vi "Sub VI TimeTest.vi"() -> ()   [LabVIEW 2021]
panel:
  out "ms / Cycle":dbl format="%.4f"
  in  "# Iterations":u32=10000
  in  "Device":T1(ring)
  in  "Instrument Address":refnum<visa-resource-name>
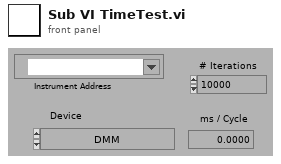
[diagram p1: front panel]
types:
  T1 = enum16{"DMM", "Keithley 2000", "HP 34401", "Memory Stats", "polynomial eval", "Null SubVI"}
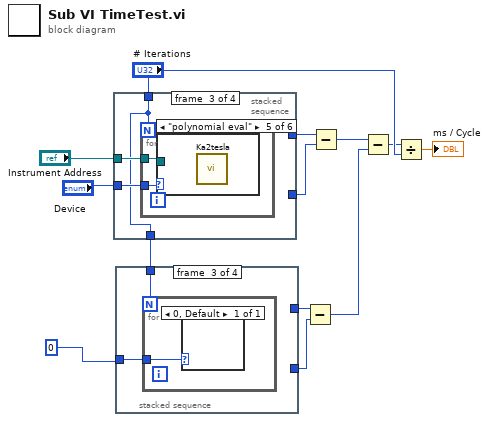
[diagram p0: block diagram]
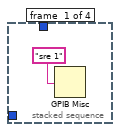
[diagram p2: hidden frame]
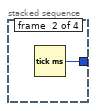
[diagram p3: hidden frame]
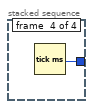
[diagram p4: hidden frame]
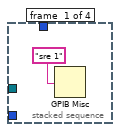
[diagram p5: hidden frame]
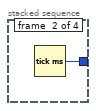
[diagram p6: hidden frame]
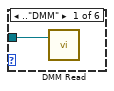
[diagram p7: hidden frame]
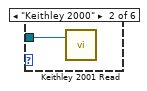
[diagram p8: hidden frame]
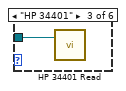
[diagram p9: hidden frame]
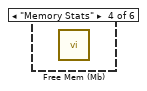
[diagram p10: hidden frame]
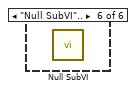
[diagram p11: hidden frame]
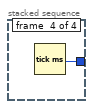
[diagram p12: hidden frame]
diagram:
  n1 = stacked-sequence {
    tunnel: "Instrument Address" -> [_ _ w18 _]
    tunnel: "Device" -> [_ _ w17 _]
    tunnel: "# Iterations" -> [_ _ w16 _]
    tunnel: [_ _ _ w24] -> w10
    tunnel: [_ w15 _ _] -> w9
    tunnel: [_ _ w16 _] -> w6
    frame #0 {
      n2 = GPIB Misc(0:"sre 1") -> ()  [unwired: 1 in, 3 out]
    }
    frame #1 {
      n3 = Tick Count (ms)() -> (millisecond timer value=w15:u32)
    }
    frame #2 {
      n4 = for {
        N: w16 -> [_]
        tunnel: w18 -> [w20]
        tunnel: w17 -> [w19]
        n5 = case shown="\"polynomial eval\"" w19 {
          tunnel: w20 -> [w21 w22 w23 _ _ _]
          frame .."DMM" {
            n6 = call "DMM Read.vi"("Instrument Address"=w21) -> ()  [unwired: 1 in, 2 out]
          }
          frame "Keithley 2000" {
            n7 = call "Keithley 2001 Read.vi"("Instrument Address"=w22) -> ()  [unwired: 1 in, 2 out]
          }
          frame "HP 34401" {
            n8 = call "HP 34401 Read.vi"("Instrument Address"=w23) -> ()  [unwired: 1 in, 2 out]
          }
          frame "Memory Stats" {
            n9 = call "Free Mem (Mb).vi"() -> ()  [unwired: 1 out]
          }
          frame "polynomial eval" {
            n10 = call "Ka2tesla.vi"() -> ()  [unwired: 2 in, 1 out]
          }
          frame "Null SubVI".. {
            n11 = call "Null SubVI.vi"() -> ()  [unwired: 1 in]
          }
        }
      }
    }
    frame #3 {
      n12 = Tick Count (ms)() -> (millisecond timer value=w24:u32)
    }
  }
  n13 = stacked-sequence {
    tunnel: 0 -> [_ _ w28 _]
    tunnel: w6 -> [_ _ w27 _]
    tunnel: [_ _ _ w30] -> w3
    tunnel: [_ w26 _ _] -> w2
    frame #0 {
      n14 = GPIB Misc(0:"sre 1") -> ()  [unwired: 1 in, 3 out]
    }
    frame #1 {
      n15 = Tick Count (ms)() -> (millisecond timer value=w26:u32)
    }
    frame #2 {
      n16 = for {
        N: w27 -> [_]
        tunnel: w28 -> [w29]
        n17 = case shown="0, Default" w29 {
          frame 0, Default {
          }
        }
      }
    }
    frame #3 {
      n18 = Tick Count (ms)() -> (millisecond timer value=w30:u32)
    }
  }
  n19 = Subtract(x=w3, y=w2) -> (x-y=w1:u32)
  n20 = Subtract(x=w10, y=w9) -> (x-y=w8:u32)
  n21 = Subtract(x=w8, y=w1) -> (x-y=w4:u32)
  n22 = Divide(x=w4, y="# Iterations") -> (x/y=→"ms / Cycle":dbl)
